vi "Initialize.vi"(8 "nonempty":refnum<k4>, 9 "nonfull":refnum<k4>, 11 "PipeData in":refnum<class "StreamData.lvclass">) -> (3 "PipeData out":refnum<class "StreamData.lvclass">)   [LabVIEW 2017, in "Stream-t'WPI_EncoderType.ctl'.lvlib" / "StreamData.lvclass"]
uses:
  <extravilib>/ChannelInstances/Stream-t'WPI_EncoderType.ctl'/StreamData.lvclass
  <resource>/ChannelSupport/_ChannelSupport/PipeLogic/PipeLogic.lvclass/PipeLogic.ctl
  <vilib>/Rock Robotics/WPI/Encoder/WPI_EncoderType.ctl
  <extravilib>/ChannelInstances/Stream-t'WPI_EncoderType.ctl'/StreamData.lvclass/StreamData.ctl
  <resource>/ChannelSupport/_ChannelSupport/PipeLogic/PipeLogic.lvclass
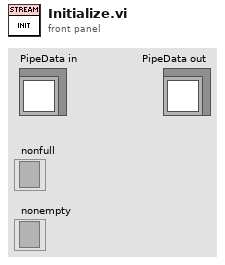
[diagram p1: front panel]
types:
  T1 = typedef "WPI_EncoderType.ctl" = enum16{"1x", "2x", "4x"}
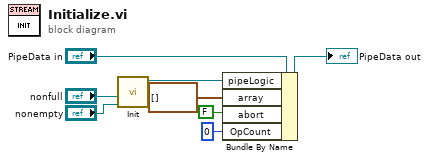
[diagram p0: block diagram]
diagram:
  n1 = call <resource>:"Init.vi"("nonEmpty"="nonempty", "nonFull"="nonfull") -> ("pipeLogic out"=w2:refnum<class "PipeLogic.lvclass">)  [unwired: 9 in]
  n2 = Bundle By Name(cluster="PipeData in", "pipeLogic"=w2, "array"=cluster{"element":T1}[] [], "abort"=FALSE, "OpCount"=u32 0) -> (→"PipeData out":refnum<class "StreamData.lvclass">)
